vi "BNC555.HandleError.vi"(0 "i ref in":refnum<vi>, 2 "Device error":errorcluster, 5 "error in (no error)":errorcluster) -> (14 "i ref out":refnum<vi>, 19 "error out":errorcluster)   [LabVIEW 2014, in "BNC555.lvlib"]
doc: "This VI handles a device error in case of any hardware communication failure. It sets the GUI element and in case of an error the dim published status to 3: failure."
uses:
  BNC555.lvlib
  CS_PHELIX/PH_Basics/PH_StatusHandler/PH_StatusHandler.Status.ctl
  CS_PHELIX/PH_Basics/PH_StatusHandler/PH_StatusHandler.lvlib
  CS_PHELIX/PH_Basics/PH_Common/PH_Common.lvlib
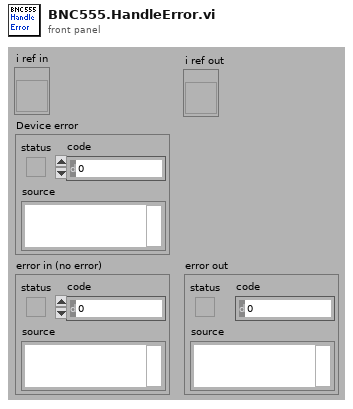
[diagram p1: front panel]
types:
  T1 = typedef "BNC555.lvlib/BNC555.i attribute.ctl" = cluster{"Information":cluster{"VISA resource name":refnum<visa-resource-name>, "Baud Rate (1:9600)":u16}, "Channel Array":T2[], "System":T3, "GUI Refs":cluster{"Delete":refnum<vi>, "Information":refnum<vi>, "System":refnum<vi>, "Channel Array":refnum<vi>, "Device Error":refnum<vi>, "Instr Driver Revision":refnum<vi>, "Instr Firmware Revision":refnum<vi>, "Instr Option":refnum<vi>, "Self-Test Response":refnum<vi>}, "Service IDs Channelinfo":i32[], "Service ID T0 Mode":i32}
  T2 = typedef "BNC555 - Driver np.lvlib/BNC555 All Chan Parameters.ctl" = cluster{"Chan #":i32, "Chan State":bool, "Chan Delay":dbl, "Chan Width":dbl, "Chan Mode":enum16{"Normal", "Single", "Burst", "Divide by N"}, "Chan Burst #":u32, "Chan Divide #":u32, "Chan Pol Out":enum16{"Normal", "Complement", "Inverted"}, "Chan Level Out":enum16{"TTL", "Adjustable", "35 Volt"}, "Chan Lev Adjust":dbl, "Chan Gate Pol":enum16{"Normal", "Complement", "Inverted"}, "Chan Gate State":bool}
  T3 = typedef "BNC555 - Driver np.lvlib/BNC555 All Sys Parameters.ctl" = cluster{"Sys Period":dbl, "Sys Oscillator":bool, "Sys Mode":enum16{"Normal", "Single", "Burst", "Duty Cycle"}, "Sys Burst #":u32, "Sys DC On":u32, "Sys DC Off":u32, "Sys Trig Mode":enum16{"Disabled", "Triggered", "Gated"}, "Sys Trig Lev":dbl, "Sys Gate State":bool, "Sys Trig Edge":bool, "Sys State":bool}
  T4 = typedef "PH_StatusHandler.lvlib/PH_StatusHandler.Status.ctl" = i16
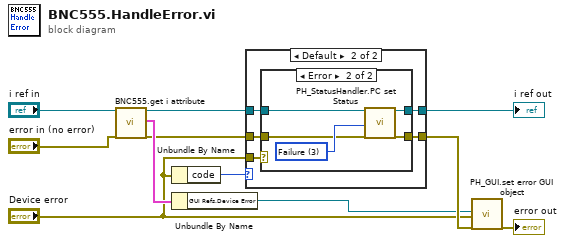
[diagram p0: block diagram]
diagram:
  n1 = call "BNC555.get i attribute.vi"("i ref in"="i ref in", "error in (no error)"="error in (no error)") -> ("i ref out"=w2:refnum<vi>, "i attribute"=w9:T1, "error out"=w7:errorcluster)  [unwired: 15 in]
  n2 = Unbundle By Name("Device error") -> ("code"=w4:i32)
  n3 = Unbundle By Name(w9) -> ("GUI Refs.Device Error"=w3:refnum<vi>)
  n4 = case shown="Default" w4 {
    tunnel: [w13 w18] -> w8
    tunnel: w7 -> [w13 w17]
    tunnel: "Device error" -> [_ w16]
    tunnel: w2 -> [w12 w15]
    tunnel: [w12 w14] -> w1
    frame -1300 {
    }
    frame Default {
      n5 = case shown="Error" w16 {
        tunnel: [w20 w25] -> w18
        tunnel: w17 -> [w20 w23]
        tunnel: w15 -> [w19 w22]
        tunnel: [w19 w21] -> w14
        frame No Error {
        }
        frame Error {
          w24 = T4 3 items=["no info", "off/false/out", "on/true/in", "Failure", "Alarm", "Status 1", "Status 2", "Status 3"] ("Status")
          n6 = call "PH_StatusHandler.PC set Status.vi"("i ref in"=w22, "Status"=w24, "error in (no error)"=w23) -> ("i ref out"=w21:refnum<vi>, "error out"=w25:errorcluster)  [unwired: 15 in]
        }
      }
    }
  }
  "i ref out" <- w1
  n7 = call "PH_GUI.set error GUI object.vi"("GUI Refs.Device Error"=w3, "error to set"="Device error", "error in (no error)"=w8) -> ("error out"=→"error out":errorcluster)  [unwired: 16 in]
